vi "RTC ini Read.vi"(0 "Firmware Backup Folder":path, 1 "error in (no error)":errorcluster) -> (2 "Description":string, 3 "Messages":string, 4 "error out":errorcluster)   [LabVIEW 2018]
uses:
  <vilib>/Utility/config.llb/Read Key (String).vi
  <vilib>/Utility/config.llb/NI_LVConfig.lvlib
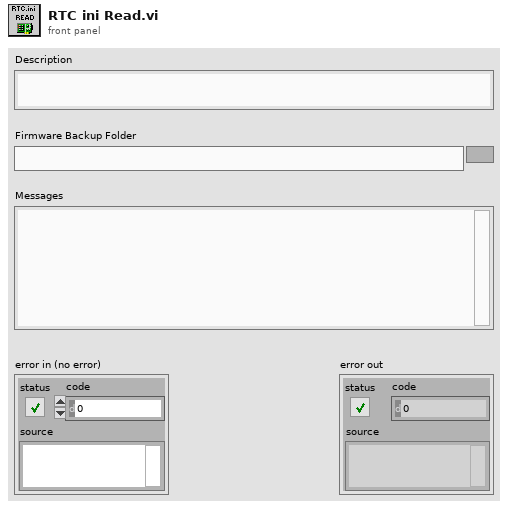
[diagram p1: front panel]
types:
  T1 = typedef "NI_LVConfig.lvlib/Config Data RefNum.ctl" = refnum<k1>
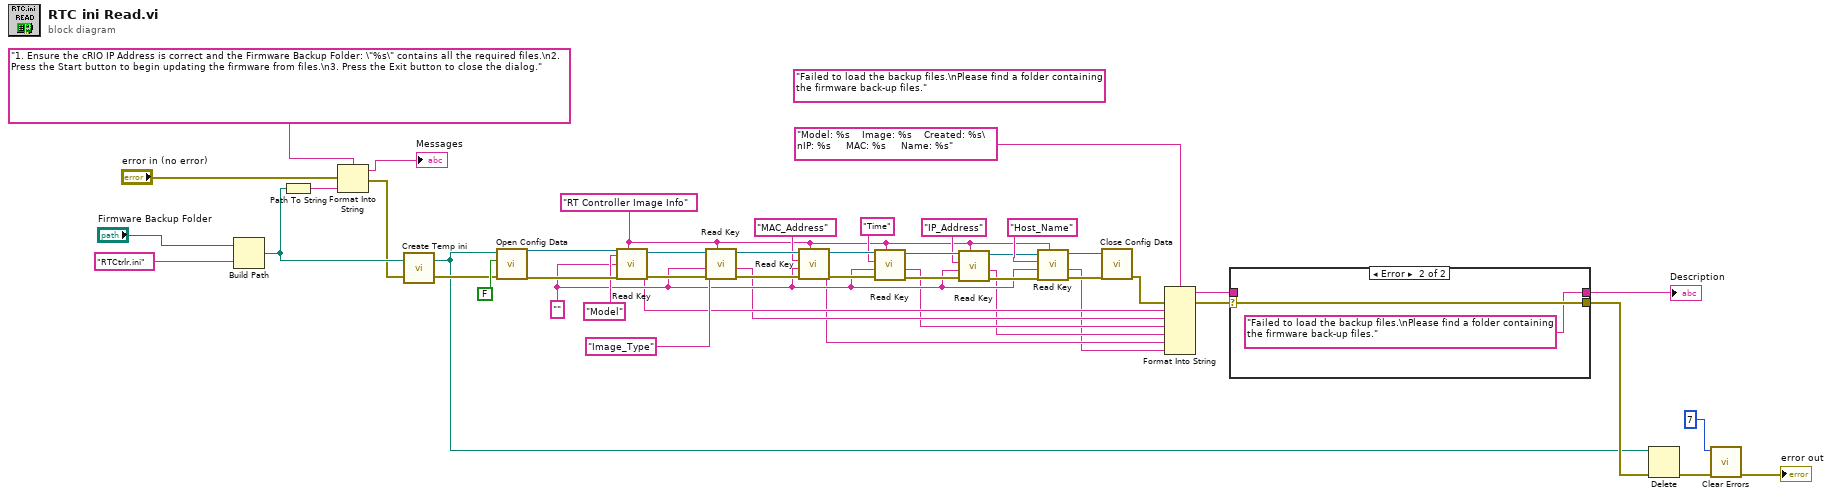
[diagram p0: block diagram]
diagram:
  (unwired) "Failed to load the backup files.\nPlease find a folder containing the firmware back-up files." ("t")
  w27 = ""
  w17 = "RT Controller Image Info" ("section")
  n1 = Build Path(base path="Firmware Backup Folder", name or relative path="RTCtrlr.ini") -> (appended path=w8:path)
  n2 = Path To String(path=w8) -> (string=w16:string)
  n3 = Format Into String(format string="1. Ensure the cRIO IP Address is correct and the Firmware Backup Folder: \"%s\" contains all the required files.\n2. Press the Start button to begin updating the firmware from files.\n3. Press the Exit button to close the dialog." ("t"), error in="error in (no error)", w16) -> (resulting string=→"Messages":string, error out=w7:errorcluster)  [unwired: 1 in]
  n4 = call "Create Temp ini.vi"("error in"=w7, "Original ini path"=w8) -> ("error out"=w6:errorcluster, "Temp ini path"=w5:path)
  n5 = call <vilib>:"Open Config Data.vi"("error in (no error)"=w6, "create file if necessary (T)"=FALSE ("create file if necessary? (T)"), "configuration file path"=w5) -> ("error out"=w46:errorcluster, "refnum"=w47:T1)  [unwired: 6 in, 1 out]
  n6 = call-poly <vilib>:"Read Key.vi"("section"=w17, "error in (no error)"=w46, "default value"=w27, "key"="Model", "refnum"=w47) -> ("error out"=w43:errorcluster, "value"=w25:string, "refnum out"=w44:T1)  [unwired: 1 in, 3 out]
  n7 = call-poly <vilib>:"Read Key.vi"("section"=w17, "error in (no error)"=w43, "default value"=w27, "key"="Image_Type", "refnum"=w44) -> ("error out"=w40:errorcluster, "value"=w24:string, "refnum out"=w41:T1)  [unwired: 1 in, 3 out]
  n8 = call-poly <vilib>:"Read Key.vi"("section"=w17, "error in (no error)"=w40, "default value"=w27, "key"="MAC_Address", "refnum"=w41) -> ("error out"=w36:errorcluster, "value"=w21:string, "refnum out"=w37:T1)  [unwired: 1 in, 3 out]
  n9 = call-poly <vilib>:"Read Key.vi"("section"=w17, "error in (no error)"=w36, "default value"=w27, "key"="Time", "refnum"=w37) -> ("error out"=w30:errorcluster, "value"=w23:string, "refnum out"=w31:T1)  [unwired: 1 in, 3 out]
  n10 = call-poly <vilib>:"Read Key.vi"("section"=w17, "error in (no error)"=w30, "default value"=w27, "key"="IP_Address", "refnum"=w31) -> ("error out"=w28:errorcluster, "value"=w22:string, "refnum out"=w29:T1)  [unwired: 1 in, 3 out]
  n11 = call-poly <vilib>:"Read Key.vi"("section"=w17, "error in (no error)"=w28, "default value"=w27, "key"="Host_Name", "refnum"=w29) -> ("error out"=w34:errorcluster, "value"=w20:string, "refnum out"=w35:T1)  [unwired: 1 in, 3 out]
  n12 = call <vilib>:"Close Config Data.vi"("error in (no error)"=w34, "refnum"=w35) -> ("error out"=w14:errorcluster)  [unwired: 1 in, 8 out]
  n13 = Format Into String(format string="Model: %s    Image: %s    Created: %s\nIP: %s     MAC: %s     Name: %s", error in=w14, w25, w24, w23, w22, w21, w20) -> (resulting string=w12:string, error out=w13:errorcluster)  [unwired: 1 in]
  n14 = case shown="Error" w13 {
    selector: w13 -> [w49 w52]
    tunnel: [w49 w52] -> w11
    tunnel: w12 -> [w50 _]
    tunnel: [w50 "Failed to load the backup files.\nPlease find a folder containing the firmware back-up files." ("t")] -> w4
    frame No Error {
    }
    frame Error {
    }
  }
  "Description" <- w4
  n15 = Delete(path (use dialog)=w5, error in=w11) -> (error out=w3:errorcluster)  [unwired: 3 in, 2 out]
  n16 = call <vilib>:"Clear Errors.vi"("error in (no error)"=w3, "specific error code to clear (0: all)"=7) -> ("error out"=→"error out":errorcluster)  [unwired: 4 in, 1 out]
